vi "GetFAMM.lvclass.vi"(8 "error in (no error)":errorcluster, 11 "HISW in":refnum<class "HISW.lvclass">) -> (0 "error out":errorcluster, 2 "FAMM.lvclass":refnum<class "FAMM.lvclass">, 3 "HISW out":refnum<class "HISW.lvclass">)   [LabVIEW 2020, in "HISW.lvclass"]
doc: "Get FAMM class object"
uses:
  HISW.lvclass
  FAMM/FAMM.lvclass
  HISW.lvclass/HISW.ctl
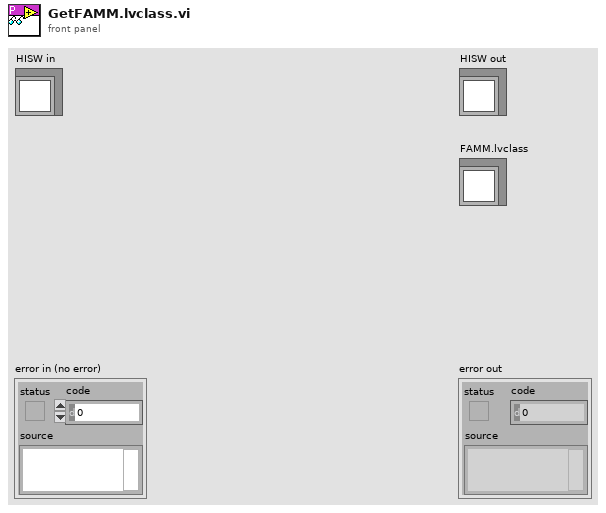
[diagram p1: front panel]
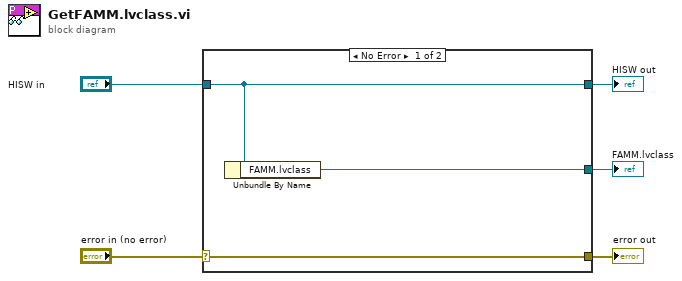
[diagram p0: block diagram]
diagram:
  n1 = case shown="No Error" "error in (no error)" {
    selector: "error in (no error)" -> [w8 w9]
    tunnel: [w8 w9] -> w4
    tunnel: [w7 w10] -> w2
    tunnel: "HISW in" -> [w7 w10]
    tunnel: [w6 _] -> w1
    frame No Error {
      n2 = Unbundle By Name(w7) -> ("FAMM.lvclass"=w6:refnum<class "FAMM.lvclass">)
    }
    frame Error {
    }
  }
  "error out" <- w4
  "HISW out" <- w2
  "FAMM.lvclass" <- w1
